vi "Cannon Modifications.vi"(1 "Cannon Global Data In":T2) -> (0 "Cannon Global Data Out":T2)   [LabVIEW 2013]
uses:
  <vilib>/Rock Robotics/WPI/Solenoid/WPI_SolenoidValue.ctl
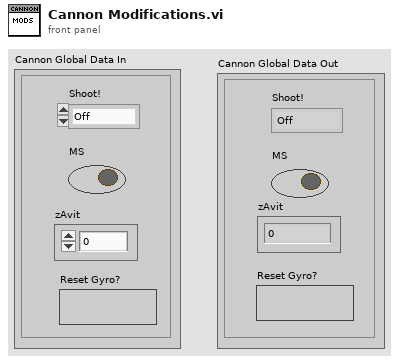
[diagram p1: front panel]
types:
  T1 = typedef "WPI_SolenoidValue.ctl" = enum16{"Off", "On", "Forward", "Reverse"}
  T2 = cluster{"MS":bool, "Shoot!":T1, "zAvit":dbl, "Reset Gyro?":bool}
  T3 = typedef "WPI_GyroDevRef.ctl" = cluster{"DevStatus":errorcluster, "Analog Module":T4, "Analog Channel":T5, "Offset":dbl, "Gain (VoltsPerDegree/Second)":dbl}
  T4 = typedef "FPGA_TypedefAnalogModule.ctl" = enum16{"Analog Module 1", "Analog Module 2"}
  T5 = typedef "FPGA_AIChannel.ctl" = enum8{"AI 1", "AI 2", "AI 3", "AI 4", "AI 5", "AI 6", "AI 7", "AI 8", "Invalid"}
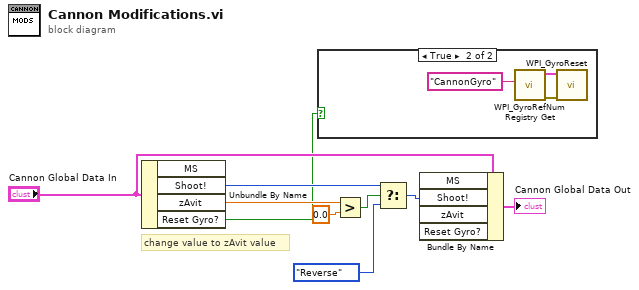
[diagram p0: block diagram]
diagram:
  # "change value to zAvit value"
  n1 = Unbundle By Name("Cannon Global Data In") -> ("Shoot!"=w2:T1, "zAvit"=w6:dbl, "Reset Gyro?"=w1:bool)  [unwired: 1 out]
  n2 = case shown="True" w1 {
    frame False {
    }
    frame True {
      n3 = call "WPI_GyroRefNum Registry Get.vi"("refnum name"="CannonGyro") -> ("error out"=w11:errorcluster, "GyroDevRef"=w10:T3)  [unwired: 9 in]
      n4 = call "WPI_GyroReset.vi"("error in (no error)"=w11, "GyroDevRef"=w10) -> ()  [unwired: 8 in, 2 out]
    }
  }
  n5 = Greater?(x=w6, y=0.0) -> (0:w4:bool)
  n6 = Select(t=w2, s=w4, f=WPI_SolenoidValue."Reverse" ("Shoot!")) -> (s? t:f=w7:T1)
  n7 = Bundle By Name(cluster="Cannon Global Data In", "Shoot!"=w7) -> (→"Cannon Global Data Out":T2)  [unwired: 3 in]
